vi "PSPara_Para Setting Operation.vi"(7 "Operation":enum16{"Set Value", "Get Value", "Initialize"}(ring)=enum."Get Value", 9 "error in (no error)":errorcluster, 10 "_Para":T1={"连续存储设置"={"Save Mode"=0, "Sel Save Mode"=0, "FolderPath"=path "", "Filename"="演示", "Explation"="演示", "AutoPoint"=0, "Template"=path ""}, "Latest Prj"=path "", "Tdms Ref*"=refnum, "默认波形图个数"=0, "列表列数"=0} {"连续存储设置"."Sel Save Mode" items=["不挑点", "自动挑点", "手动挑点"]; "连续存储设置"."Save Mode" items=["不存储", "连续存储"]}) -> (1 "error out":errorcluster, 2 "_Para":T1={"连续存储设置"={"Save Mode"=0, "Sel Save Mode"=0, "FolderPath"=path "", "Filename"="演示", "Explation"="演示", "AutoPoint"=0, "Template"=path ""}, "Latest Prj"=path "", "Tdms Ref*"=refnum, "默认波形图个数"=0, "列表列数"=0} {"连续存储设置"."Sel Save Mode" items=["不挑点", "自动挑点", "手动挑点"]; "连续存储设置"."Save Mode" items=["不存储", "连续存储"]})   [LabVIEW 2016]
uses:
  Controls/Global para Config.ctl
panel:
  # "SampleMode断开了自定义类型连接"
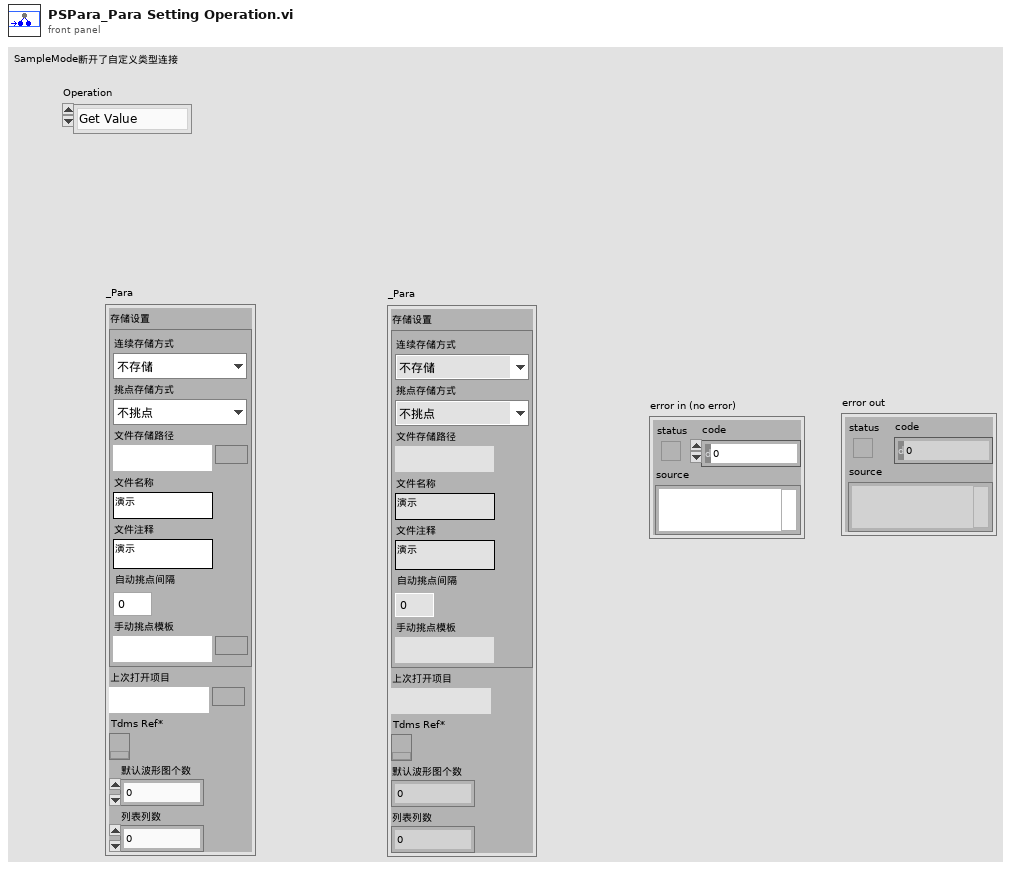
[diagram p1: front panel]
types:
  T1 = typedef "Global para Config.ctl" = cluster{"连续存储设置":cluster{"Save Mode":i32, "Sel Save Mode":i32, "FolderPath":path, "Filename":string, "Explation":string, "AutoPoint":i32, "Template":path}, "Latest Prj":path, "Tdms Ref*":refnum<k34>, "默认波形图个数":u8, "列表列数":u8}
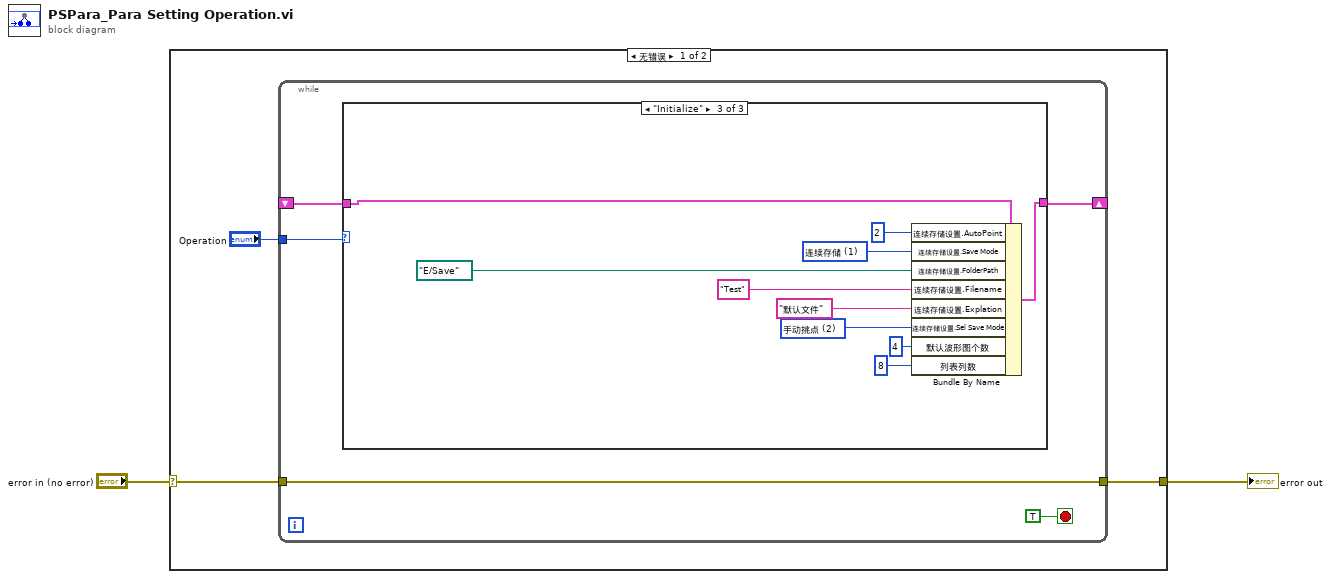
[diagram p0: block diagram]
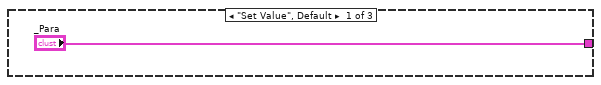
[diagram p2: hidden frame]
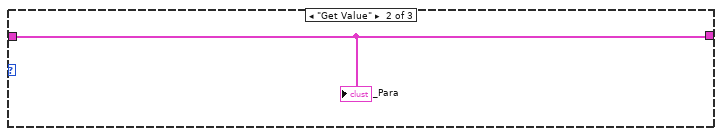
[diagram p3: hidden frame]
diagram:
  n1 = case shown="无错误" "error in (no error)" {
    selector: "error in (no error)" -> [w4 w23]
    tunnel: [w3 w23] -> w1
    frame No Error {
      n2 = while {
        tunnel: "Operation" -> [w9]
        shift-right: [w8] -> _
        shift-left: _ -> [w7]
        tunnel: w4 -> [w6]
        tunnel: [w6] -> w3
        stop <- TRUE stop-if-true
        n3 = case shown="\"Initialize\"" w9 {
          tunnel: ["_Para" w12 w21] -> w8
          tunnel: w7 -> [_ w12 w22]
          frame "Set Value", Default {
          }
          frame "Get Value" {
            "_Para" <- w12
          }
          frame "Initialize" {
            w18 = 1 items=["不存储", "连续存储"] ("Save Mode")
            w19 = 2 items=["不挑点", "自动挑点", "手动挑点"] ("Save Mode")
            n4 = Bundle By Name(cluster=w22, "连续存储设置.AutoPoint"=2 ("存储设置.AutoPoint"), "连续存储设置.Save Mode"=w18, "连续存储设置.FolderPath"=path "E:/Save", "连续存储设置.Filename"="Test" ("Save.Filename"), "连续存储设置.Explation"="默认文件" ("Save.Explation"), "连续存储设置.Sel Save Mode"=w19, "默认波形图个数"=u8 4, "列表列数"=u8 8) -> (w21:T1)
          }
        }
      }
    }
    frame Error {
    }
  }
  "error out" <- w1
